vi "硬盘剩余空间查询.vi"() -> (1 "磁盘曝光时间(str)":string, 2 "磁盘剩余空间不够":bool, 3 "磁盘剩余(G)":u64)   [LabVIEW 2014]
uses:
  Global.vi
panel:
  out "无符号64位整型":u64
  out "数字":u64
  out "子字符串之后":string
  out "standard output":string caption="标准输出"
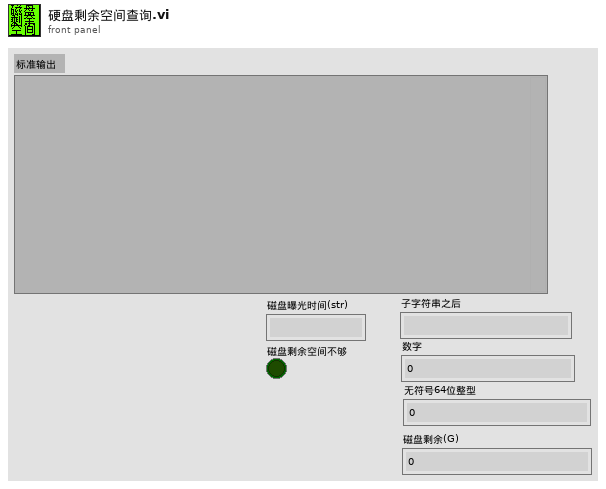
[diagram p1: front panel]
types:
  T1 = typedef "OtherSpec.ctl" = cluster{"其它勾选类规格":T2, "其它数据类规格":T3, "相机名称":T4, "参数":cluster{"Mark1曝光时间":i32, "Mark2曝光时间":i32, "二维码曝光时间":i32}}
  T2 = typedef "其它勾选类规格.ctl" = cluster{"保存图片":bool, "上传设备状态数据":bool, "保存数据":bool, "开机默认开启监控摄像头":bool, "启用mark拍照 ":bool}
  T3 = typedef "其他数据类规格.ctl" = cluster{"相机1像素-毫米换算系数":dbl, "相机2像素-毫米换算系数":dbl, "D盘剩余空间预警(G)":dbl, "视频最长录制时间(秒)":dbl}
  T4 = typedef "相机名称品牌使用状态.ctl" = cluster{"相机1名称":T5, "相机2名称":T5, "Cam1启用":bool, "Cam2启用":bool, "Basler1":bool, "Basler2":bool}
  T5 = typedef "IMAQdx.ctl" = refnum<k21>
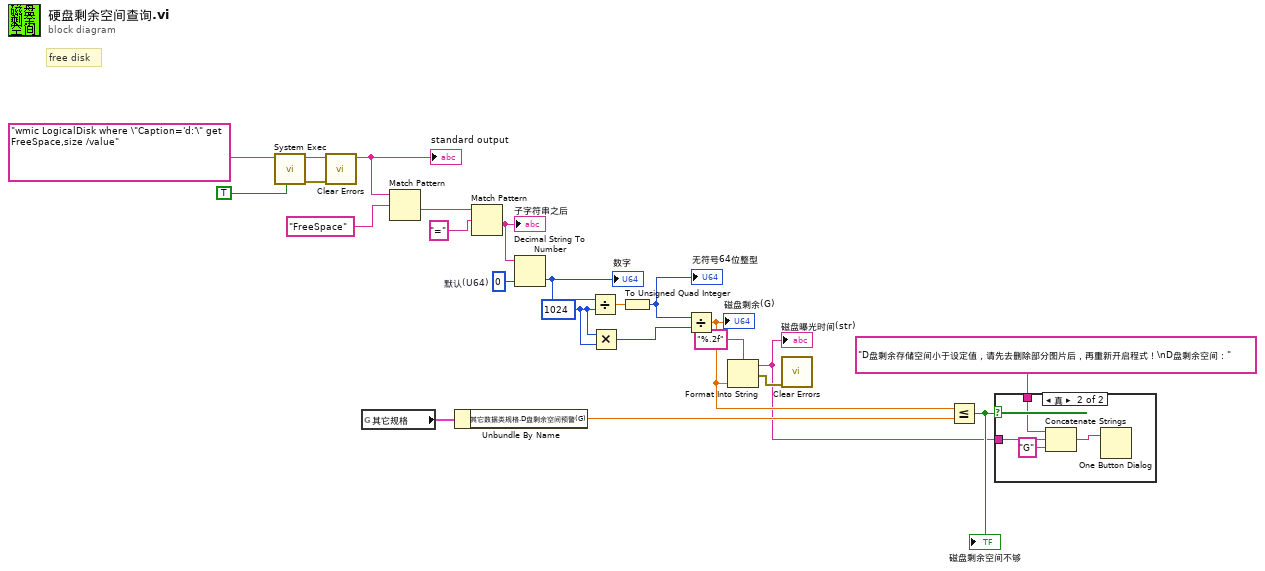
[diagram p0: block diagram]
diagram:
  w14 = u64 0  # 默认(U64)
  w10 = u64 1024 ("y")
  # "free disk"
  n1 = call <vilib>:"System Exec.vi"("run minimized? (F)"=TRUE, "command line"="wmic LogicalDisk where \"Caption='d:'\" get FreeSpace,size /value" ("字符串")) -> ("error out"=w13:errorcluster, "standard output"=w20:string)  [unwired: 6 in, 2 out]
  "standard output" <- w20
  n2 = call <vilib>:"Clear Errors.vi"("error in (no error)"=w13) -> ()  [unwired: 5 in, 2 out]
  n3 = global read "Global.vi" "其它规格"() -> (w7:T1)
  n4 = Match Pattern(string=w20, regular expression="FreeSpace" ("搜索字符串")) -> (after substring=w18:string)  [unwired: 1 in, 3 out]
  n5 = Unbundle By Name(w7) -> ("其它数据类规格.D盘剩余空间预警(G)"=w4:dbl)
  n6 = Match Pattern(string=w18, regular expression="=" ("正则表达式")) -> (after substring=w16:string)  [unwired: 1 in, 3 out]
  "子字符串之后" <- w16
  n7 = Decimal String To Number(string=w16, default (0L)=w14) -> (number=w15:u64)  [unwired: 1 in, 1 out]
  "数字" <- w15
  n8 = Divide(x=w15, y=w10) -> (x/y=w12:dbl)
  n9 = Multiply(x=w10, y=w10) -> (x*y=w9:u64)
  n10 = To Unsigned Quad Integer(1:w12) -> (0:w11:u64)
  "无符号64位整型" <- w11
  n11 = Divide(x=w11, y=w9) -> (x/y=w3:dbl)
  "磁盘剩余(G)" <- w3
  n12 = Format Into String(format string="%.2f" ("格式字符串"), w3) -> (resulting string=w2:string, error out=w8:errorcluster)  [unwired: 2 in]
  "磁盘曝光时间(str)" <- w2
  n13 = call <vilib>:"Clear Errors.vi"("error in (no error)"=w8) -> ()  [unwired: 5 in, 2 out]
  n14 = Less Or Equal?(x=w3, y=w4) -> (x <= y?=w5:bool)
  "磁盘剩余空间不够" <- w5
  n15 = case shown="真" w5 {
    tunnel: "D盘剩余存储空间小于设定值，请先去删除部分图片后，再重新开启程式！\nD盘剩余空间：" -> [_ w26]
    tunnel: w2 -> [_ w24]
    frame False {
    }
    frame True {
      n16 = Concatenate Strings(w26, w24, "G" ("字符串")) -> (w25:string)
      n17 = One Button Dialog(message=w25) -> ()  [unwired: 1 in, 1 out]
    }
  }
